vi "ReportLocalPose.vi"(1 "Destination":T3={"Subsystem Id"=90, "Node Id"=1, "Component Id"=1}, 2 "PresenceVector":u16=2 format="%b", 3 "LocalPose":T1, 4 "Source":T3={"Subsystem Id"=3, "Node Id"=1, "Component Id"=1}) -> (0 "Encoded JAUS Message":string)   [LabVIEW 2009]
uses:
  Support Files/Address.ctl
  Support Files/LocalPose.ctl
  Support Files/TimeRec.ctl
panel:
  in  "Current Time":bool
  in  "Command Code":string="D\u0003"
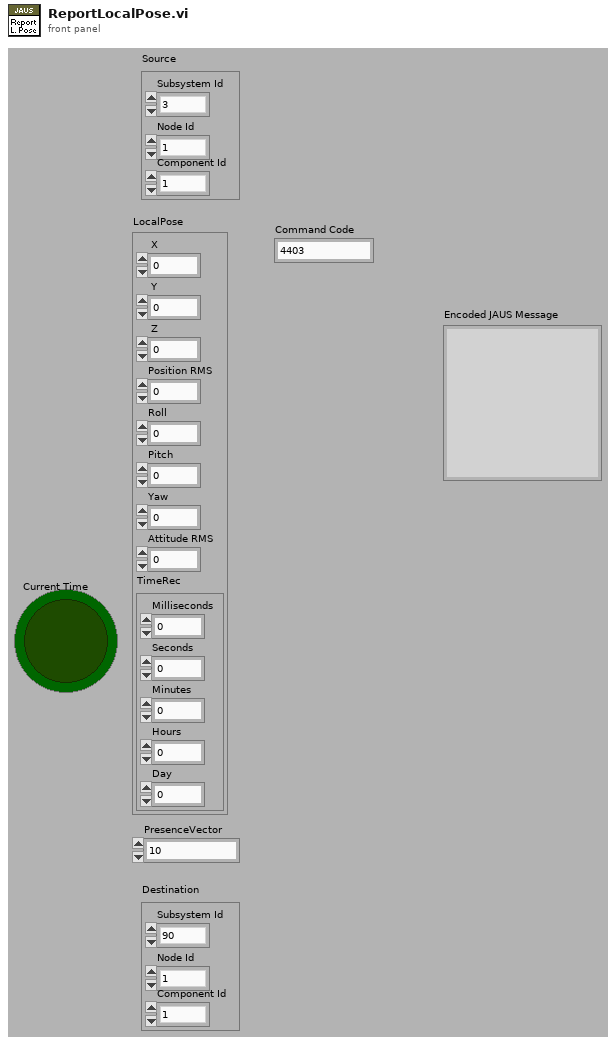
[diagram p1: front panel]
types:
  T1 = typedef "LocalPose.ctl" = cluster{" X":dbl, " Y":dbl, " Z":dbl, "Position RMS":dbl, "Roll":dbl, "Pitch":dbl, "Yaw":dbl, "Attitude RMS":dbl, "TimeRec":T2}
  T2 = typedef "TimeRec.ctl" = cluster{"Milliseconds":u32, "Seconds":u32, "Minutes":u32, "Hours":u32, "Day":u32}
  T3 = typedef "Address.ctl" = cluster{"Subsystem Id":u16, "Node Id":u8, "Component Id":u8}
  T4 = cluster{"unsigned byte array[0]":u8, "unsigned byte array[1]":u8}
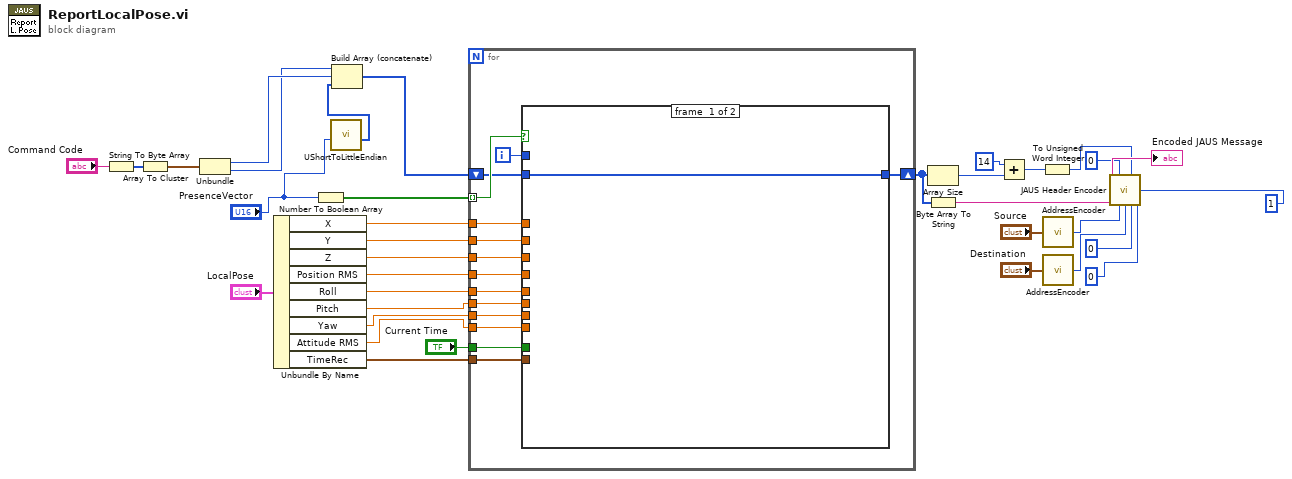
[diagram p0: block diagram]
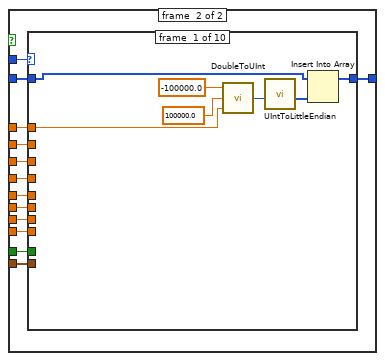
[diagram p2: hidden frame]
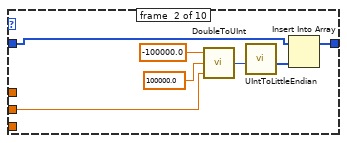
[diagram p3: hidden frame]
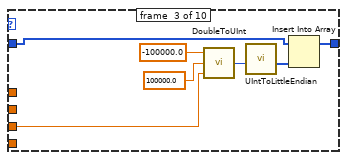
[diagram p4: hidden frame]
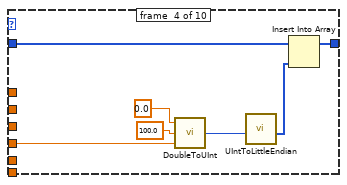
[diagram p5: hidden frame]
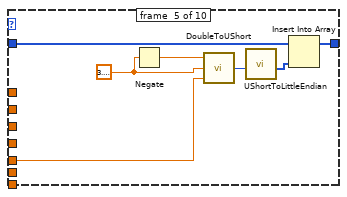
[diagram p6: hidden frame]
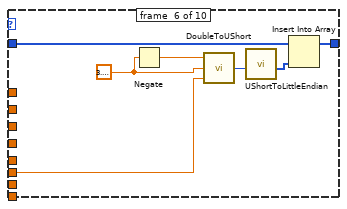
[diagram p7: hidden frame]
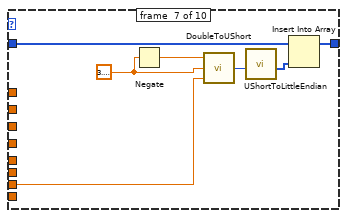
[diagram p8: hidden frame]
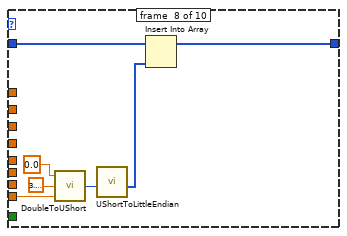
[diagram p9: hidden frame]
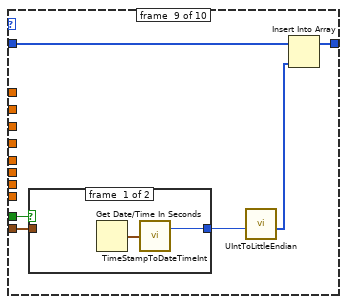
[diagram p10: hidden frame]
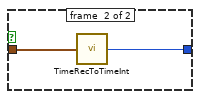
[diagram p11: hidden frame]
diagram:
  n1 = String To Byte Array(string="Command Code") -> (unsigned byte array=w12:u8[])
  n2 = Array To Cluster(array=w12) -> (cluster=w11:T4)
  n3 = Unbundle(w11) -> ("unsigned byte array[0]"=w10:u8, "unsigned byte array[1]"=w9:u8)
  n4 = Unbundle By Name("LocalPose") -> ("X"=w22:dbl, "Y"=w21:dbl, "Z"=w20:dbl, "Position RMS"=w19:dbl, "Roll"=w18:dbl, "Pitch"=w17:dbl, "Yaw"=w16:dbl, "Attitude RMS"=w15:dbl, "TimeRec"=w14:T2)
  n5 = Number To Boolean Array(number="PresenceVector") -> (Boolean array=w26:bool[])
  n6 = call "UShortToLittleEndian.vi"("Number"="PresenceVector") -> ("byte array"=w1:u8[])  [unwired: 10 in]
  n7 = Build Array (concatenate)(w9, w10, w1) -> (w8:u8[])
  n8 = for {
    tunnel: w26 -> [w49] mode=indexing
    tunnel: w22 -> [w47]
    tunnel: w21 -> [w46]
    tunnel: w20 -> [w45]
    tunnel: w19 -> [w44]
    tunnel: w18 -> [w43]
    tunnel: w17 -> [w42]
    tunnel: w16 -> [w41]
    tunnel: w15 -> [w40]
    tunnel: w14 -> [w39]
    shift-right: [w38] -> w4
    shift-left: w8 -> [w37]
    tunnel: "Current Time" -> [w36]
    i -> [w48]
    n9 = case shown="False" w49 {
      tunnel: w48 -> [_ w63]
      tunnel: w47 -> [_ w62]
      tunnel: w46 -> [_ w61]
      tunnel: w45 -> [_ w60]
      tunnel: w44 -> [_ w59]
      tunnel: w43 -> [_ w58]
      tunnel: w42 -> [_ w57]
      tunnel: w41 -> [_ w56]
      tunnel: w40 -> [_ w55]
      tunnel: w39 -> [_ w54]
      tunnel: [w50 w53] -> w38
      tunnel: w37 -> [w50 w52]
      tunnel: w36 -> [_ w51]
      frame #0 {
      }
      frame #1 {
        n10 = case shown="Default" w63 {
          tunnel: w62 -> [w66 _ _ _ _ _ _ _ _ _]
          tunnel: w61 -> [_ w73 _ _ _ _ _ _ _ _]
          tunnel: w60 -> [_ _ w80 _ _ _ _ _ _ _]
          tunnel: w59 -> [_ _ _ w87 _ _ _ _ _ _]
          tunnel: w58 -> [_ _ _ _ w96 _ _ _ _ _]
          tunnel: w57 -> [_ _ _ _ _ w103 _ _ _ _]
          tunnel: w56 -> [_ _ _ _ _ _ w110 _ _ _]
          tunnel: w55 -> [_ _ _ _ _ _ _ w116 _ _]
          tunnel: w54 -> [_ _ _ _ _ _ _ _ w124 _]
          tunnel: [w65 w71 w79 w86 w92 w100 w106 w113 w121 w130] -> w53
          tunnel: w52 -> [w64 w72 w78 w85 w93 w99 w107 w114 w122 w130]
          tunnel: w51 -> [_ _ _ _ _ _ _ _ w120 _]
          frame #0 {
            n11 = call "DoubleToUInt.vi"("Value"=w66, "Max"=100000.0, "Min"=-100000.0) -> ("scaled Integer"=w68:u32)
            n12 = call "UIntToLittleEndian.vi"("Number"=w68) -> ("byte array"=w67:u8[])  [unwired: 10 in]
            n13 = Insert Into Array(array=w64, new element=w67) -> (w65:u8[])  [unwired: 1 in]
          }
          frame #1 {
            n14 = call "DoubleToUInt.vi"("Value"=w73, "Max"=100000.0, "Min"=-100000.0) -> ("scaled Integer"=w75:u32)
            n15 = call "UIntToLittleEndian.vi"("Number"=w75) -> ("byte array"=w74:u8[])  [unwired: 10 in]
            n16 = Insert Into Array(array=w72, new element=w74) -> (w71:u8[])  [unwired: 1 in]
          }
          frame #2 {
            n17 = call "DoubleToUInt.vi"("Value"=w80, "Max"=100000.0, "Min"=-100000.0) -> ("scaled Integer"=w82:u32)
            n18 = call "UIntToLittleEndian.vi"("Number"=w82) -> ("byte array"=w81:u8[])  [unwired: 10 in]
            n19 = Insert Into Array(array=w78, new element=w81) -> (w79:u8[])  [unwired: 1 in]
          }
          frame #3 {
            n20 = call "DoubleToUInt.vi"("Value"=w87, "Max"=100.0, "Min"=0.0) -> ("scaled Integer"=w89:u32)
            n21 = call "UIntToLittleEndian.vi"("Number"=w89) -> ("byte array"=w88:u8[])  [unwired: 10 in]
            n22 = Insert Into Array(array=w85, new element=w88) -> (w86:u8[])  [unwired: 1 in]
          }
          frame #4 {
            w94 = 3.141592653589793 ("Min")
            n23 = Negate(x=w94) -> (-x=w95:dbl)
            n24 = call "DoubleToUShort.vi"("Value"=w96, "Max"=w94, "Min"=w95) -> ("scaled Integer"=w98:u16)
            n25 = call "UShortToLittleEndian.vi"("Number"=w98) -> ("byte array"=w97:u8[])  [unwired: 10 in]
            n26 = Insert Into Array(array=w93, new element=w97) -> (w92:u8[])  [unwired: 1 in]
          }
          frame #5 {
            w101 = 3.141592653589793 ("Min")
            n27 = Negate(x=w101) -> (-x=w102:dbl)
            n28 = call "DoubleToUShort.vi"("Value"=w103, "Max"=w101, "Min"=w102) -> ("scaled Integer"=w105:u16)
            n29 = call "UShortToLittleEndian.vi"("Number"=w105) -> ("byte array"=w104:u8[])  [unwired: 10 in]
            n30 = Insert Into Array(array=w99, new element=w104) -> (w100:u8[])  [unwired: 1 in]
          }
          frame #6 {
            w108 = 3.141592653589793 ("Min")
            n31 = Negate(x=w108) -> (-x=w109:dbl)
            n32 = call "DoubleToUShort.vi"("Value"=w110, "Max"=w108, "Min"=w109) -> ("scaled Integer"=w112:u16)
            n33 = call "UShortToLittleEndian.vi"("Number"=w112) -> ("byte array"=w111:u8[])  [unwired: 10 in]
            n34 = Insert Into Array(array=w107, new element=w111) -> (w106:u8[])  [unwired: 1 in]
          }
          frame #7 {
            n35 = call "DoubleToUShort.vi"("Value"=w116, "Max"=3.141592653589793 ("Min"), "Min"=0.0) -> ("scaled Integer"=w118:u16)
            n36 = call "UShortToLittleEndian.vi"("Number"=w118) -> ("byte array"=w117:u8[])  [unwired: 10 in]
            n37 = Insert Into Array(array=w114, new element=w117) -> (w113:u8[])  [unwired: 1 in]
          }
          frame #8 {
            n38 = case shown="True" w120 {
              tunnel: w124 -> [_ w129]
              tunnel: [w126 w128] -> w123
              frame #0 {
                n39 = Get Date/Time In Seconds() -> (seconds since 1Jan1904=w127:timestamp)
                n40 = call "TimeStampToDateTimeInt.vi"("Time Stamp"=w127) -> ("timeInt"=w126:u32)  [unwired: 1 out]
              }
              frame #1 {
                n41 = call "TimeRecToTimeInt.vi"("TimeRec"=w129) -> ("timeInt"=w128:u32)
              }
            }
            n42 = call "UIntToLittleEndian.vi"("Number"=w123) -> ("byte array"=w125:u8[])  [unwired: 10 in]
            n43 = Insert Into Array(array=w122, new element=w125) -> (w121:u8[])  [unwired: 1 in]
          }
          frame #9 {
          }
        }
      }
    }
  }
  n44 = Array Size(array=w4) -> (size(s)=w6:i32)
  n45 = Byte Array To String(unsigned byte array=w4) -> (string=w25:string)
  n46 = Add(x=14, y=w6) -> (x+y=w5:i32)
  n47 = To Unsigned Word Integer(number=w5) -> (unsigned 16bit integer=w24:u16)
  n48 = call "AddressEncoder.vi"("Address Cluster"="Source") -> ("Address"=w34:u32)
  n49 = call "AddressEncoder.vi"("Address Cluster"="Destination") -> ("Address"=w33:u32)
  n50 = call "JAUS Header Encoder.vi"("Message Type (0-5)"=u8 0, "Data Size (8-23)"=w24, "Priority(40-41)"=u8 1, "Payload"=w25, "Source ID (80-95)"=w34, "Destination ID (48-79)"=w33, "Data Flags (46-47)"=u8 0, "Ack/Nak (44-45)"=u8 0) -> ("Encoded JAUS Message"=→"Encoded JAUS Message":string)  [unwired: 7 in]
